vi "VI_unlock.vi"(6 "Verify salt (T)":bool=TRUE, 7 "Remove lib password (T)":bool=TRUE, 8 "error in (no error)":errorcluster, 9 "New Password (\"\")":string, 10 "Output file":path, 11 "Input file":path) -> (0 "error out":errorcluster, 1 "Hash1 salt":string, 2 "Icon":picture, 3 "Version string":string, 4 "Bruteforced salt":bool)   [LabVIEW 2023]
uses:
  <vilib>/Utility/error.llb/Trim Whitespace One-Sided.vi
panel:
  # "(Disable to repair broken BDPW hashes)"
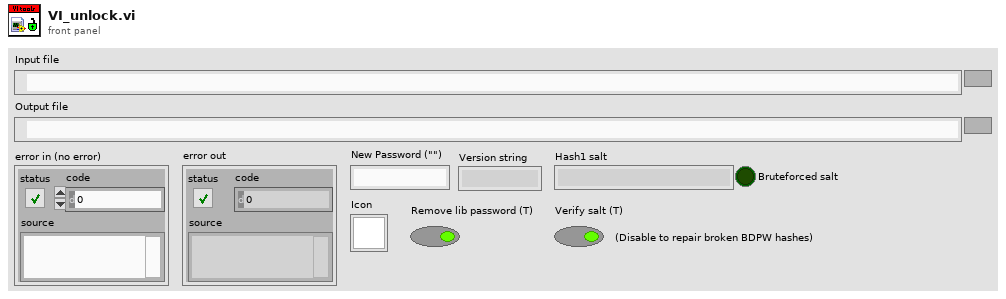
[diagram p1: front panel]
types:
  T1 = cluster{"Major":u8, "Minor":u8, "Fix":u8, "Build":u8}
  T2 = enum16{"open", "replace", "create", "open or create", "replace or create", "replace or create with confirmation"}
  T3 = map{string, cluster{"Offset":i32, "Data":string}}
  T4 = cluster{"Hash1 raw (no salt)":string, "Hash1 (MD5)":string, "VIType":u16}
  T5 = cluster{"version":u32, "Flags":u32, "viFlags2":u32, "viFlags0C":u32, "viFlags10":u32, "buttonsHidden":u16, "frontpFlags":u16, "instrState":u32, "execState":u32, "execPrio":u16, "viType":u16, "prefExecSyst":i32, "field28":u32, "field2C":u32, "field30":u32, "viSignatureHi":u64, "viSignatureLo":u64, "alignGridFP":u32, "alignGridBD":u32, "field4C":u16, "ctrlIndStyle":u16, "field50_md5Hi":u64, "field50_md5Lo":u64, "libHi":u64, "libLo":u64}
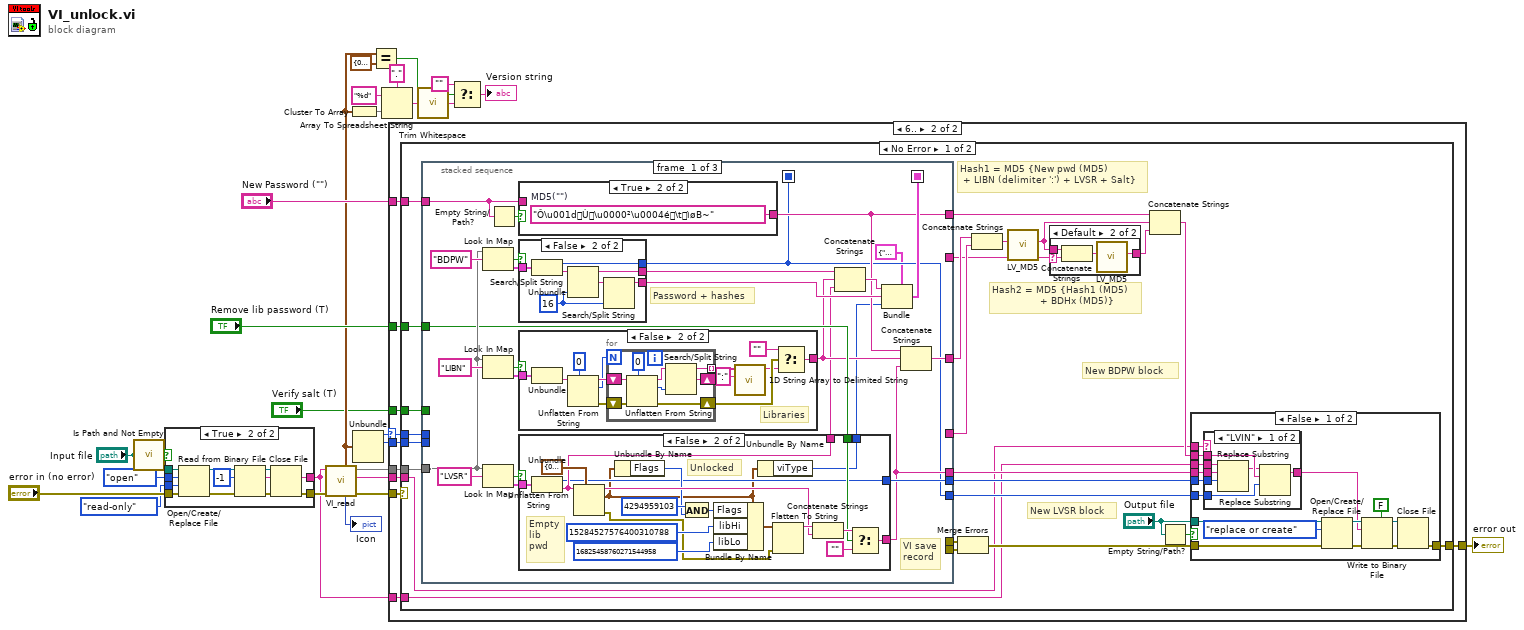
[diagram p0: block diagram]
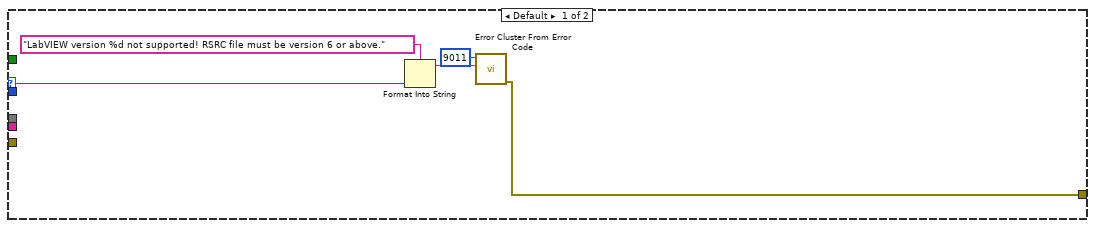
[diagram p2: hidden frame]
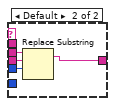
[diagram p4: hidden frame]
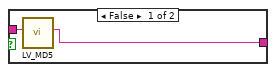
[diagram p6: hidden frame]
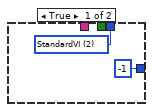
[diagram p7: hidden frame]
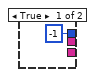
[diagram p9: hidden frame]
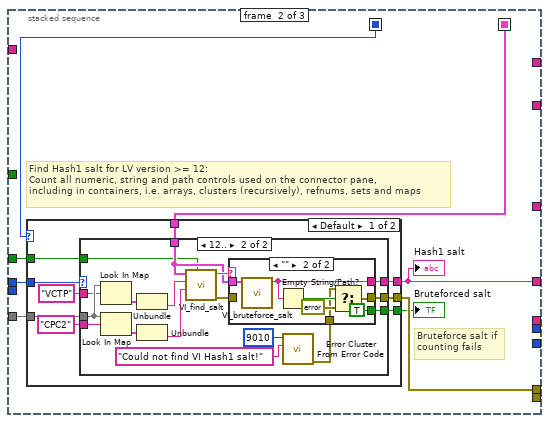
[diagram p10: hidden frame]
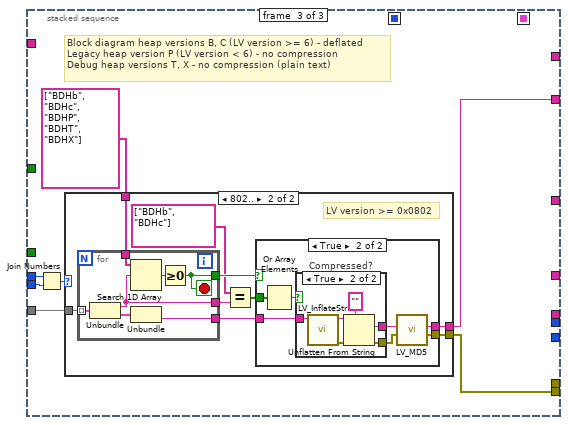
[diagram p14: hidden frame]
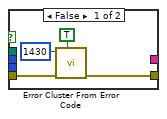
[diagram p19: hidden frame]
diagram:
  n1 = call <vilib>:"Is Path and Not Empty.vi"("path"="Input file") -> ("Is Path and Not Empty?"=w19:bool)  [unwired: 4 in]
  n2 = case "Empty?" shown="True" w19 {
    tunnel: "error in (no error)" -> [w31 w42]
    tunnel: "Input file" -> [_ w41]
    tunnel: [w28 w32] -> w27
    tunnel: enum16{"read/write", "read-only", "write-only"}."read-only" ("access (0:read/write)") -> [_ w40]
    tunnel: T2."open" ("operation (0:open)") -> [_ w39]
    tunnel: [_ w35] -> w5
    frame False {
      n3 = call <vilib>:"Error Cluster From Error Code.vi"("show call chain? (False)"=TRUE, "error in (no error)"=w31, "error code (0)"=1430) -> ("error out"=w28:errorcluster)  [unwired: 6 in]
    }
    frame True {
      n4 = Open/Create/Replace File(file path (use dialog)=w41, error in=w42, operation (0:open)=w39, access (0:read/write)=w40) -> (refnum out=w37:refnum<file>, error out=w38:errorcluster)  [unwired: 2 in, 1 out]
      n5 = Read from Binary File(8:w38, 10:-1 ("count (1)"), 11:w37) -> (0:w33:errorcluster, 2:w35:string, 3:w34:refnum<file>)  [unwired: 3 in, 1 out]
      n6 = Close File(refnum=w34, error in=w33) -> (error out=w32:errorcluster)  [unwired: 1 out]
    }
  }
  n7 = call "VI_read.vi"("error in (no error)"=w27, "File bytestream"=w5) -> ("error out"=w23:errorcluster, "Resource type"=w18:string, "Blocks"=w21:T3, "Icon"=→"Icon":picture, "Version"=w4:T1)  [unwired: 5 in]
  n8 = Cluster To Array(cluster=w4) -> (array=w12:u8[])
  n9 = Unbundle(w4) -> ("Major"=w3:u8, "Minor"=w2:u8)  [unwired: 2 out]
  n10 = Equal?(x=w4, y=T1 {"Major"=0, "Minor"=0, "Fix"=0, "Build"=0}) -> (x = y?=w10:bool)
  n11 = Array To Spreadsheet String(delimiter (Tab)=".", array=w12, 3:"%d" ("format string")) -> (spreadsheet string=w13:string)
  n12 = case shown="6.." w3 {
    selector: w3 -> [w45 w50]
    tunnel: w23 -> [_ w57]
    tunnel: [w43 w56] -> w22
    tunnel: w21 -> [_ w55]
    tunnel: w18 -> [_ w54]
    tunnel: "New Password (\"\")" -> [_ w53]
    tunnel: "Remove lib password (T)" -> [_ w52]
    tunnel: w5 -> [_ w51]
    tunnel: w2 -> [_ w49]
    tunnel: "Verify salt (T)" -> [_ w48]
    frame Default {
      n13 = Format Into String(format string="LabVIEW version %d not supported! RSRC file must be version 6 or above.", w45) -> (resulting string=w44:string)  [unwired: 2 in, 1 out]
      n14 = call <vilib>:"Error Cluster From Error Code.vi"("error message (\"\")"=w44, "error code (0)"=9011) -> ("error out"=w43:errorcluster)  [unwired: 7 in]
    }
    frame 6.. {
      n15 = case shown="No Error" w57 {
        selector: w57 -> [_ w272]
        tunnel: w55 -> [w71 _]
        tunnel: w54 -> [w61 _]
        tunnel: [w62 w272] -> w56
        tunnel: w50 -> [w66 _]
        tunnel: w53 -> [w70 _]
        tunnel: w52 -> [w69 _]
        tunnel: w51 -> [w60 _]
        tunnel: w49 -> [w59 _]
        tunnel: w48 -> [w58 _]
        frame No Error {
          # "New BDPW block"
          # "New LVSR block"
          # "Hash2 = MD5 {Hash1 (MD5)\n                + BDHx (MD5)}"
          # "Hash1 = MD5 {New pwd (MD5)\n + LIBN (delimiter ':') + LVSR + Salt}"
          n16 = stacked-sequence {
            seq-local: [w122 _ _] -> [_ w197 _]
            seq-local: [w117 _ _] -> [_ w193 _]
            tunnel: [_ w195 _] -> w76
            tunnel: w70 -> [w125 _ _]
            tunnel: [_ _ w241] -> w65
            tunnel: [w127 _ _] -> w78
            tunnel: [w120 _ _] -> w77
            tunnel: [w117 _ _] -> w64
            tunnel: [_ _ w240] -> w81
            tunnel: w71 -> [w132 w196 w239]
            tunnel: w69 -> [w128 _ _]
            tunnel: [w119 _ _] -> w68
            tunnel: [w118 _ _] -> w67
            tunnel: w66 -> [_ w199 w237]
            tunnel: [_ w198 _] -> w82
            tunnel: w59 -> [_ _ w236]
            tunnel: w58 -> [_ w192 _]
            frame #0 {
              # "VI save\nrecord"
              # "Password + hashes"
              n17 = Look In Map(map=w132, key="BDPW") -> (key not found?=w138:bool, value=w137:cluster{"Offset":i32, "Data":string})  [unwired: 1 in]
              n18 = Look In Map(map=w132, key="LIBN") -> (key not found?=w135:bool, value=w134:cluster{"Offset":i32, "Data":string})  [unwired: 1 in]
              n19 = Look In Map(map=w132, key="LVSR") -> (key not found?=w130:bool, value=w129:cluster{"Offset":i32, "Data":string})  [unwired: 1 in]
              n20 = Empty String/Path?(string/path=w125) -> (empty?=w126:bool)
              n21 = case shown="True" w126 {
                tunnel: w125 -> [w141 _]
                tunnel: [w140 w142] -> w119
                frame False {
                  n22 = call "LV_MD5.vi"("Input string"=w141) -> ("MD5 digest (16-bytes)"=w140:string)  [unwired: 9 in, 1 out]
                }
                frame True {
                  w142 = "Ô\u001dÙ\u0000²\u0004é\tìøB~"  # MD5("")
                }
              }
              n23 = case "Has BDPW?" shown="False" w138 {
                tunnel: w137 -> [_ w191]
                tunnel: [-1 ("Offset") w190] -> w117
                tunnel: [_ w186] -> w131
                tunnel: [_ w185] -> w123
                frame True {
                }
                frame False {
                  w187 = 16 ("offset (0)")
                  n24 = Unbundle(w191) -> ("Offset"=w190:i32, "Data"=w189:string)
                  n25 = Search/Split String(string=w189, offset (0)=w187) -> (substring before match=w186:string, match + rest of string=w188:string)  [unwired: 1 in, 1 out]
                  n26 = Search/Split String(string=w188, offset (0)=w187) -> (substring before match=w185:string)  [unwired: 1 in, 2 out]
                }
              }
              n27 = case "Has LIBN?" shown="False" w135 {
                tunnel: w134 -> [_ w171]
                tunnel: [_ w164] -> w121
                frame True {
                }
                frame False {
                  # "Libraries"
                  n28 = Unbundle(w171) -> ("Data"=w170:string)  [unwired: 1 out]
                  n29 = Unflatten From String(type=0 ("I32"), binary string=w170) -> (rest of the binary string=w173:string, value=w172:i32, error out=w174:errorcluster)  [unwired: 3 in]
                  n30 = for {
                    N: w172 -> [_]
                    shift-right: [w177] -> _
                    shift-left: w173 -> [w181]
                    shift-right: [w178] -> w167
                    shift-left: w174 -> [w182]
                    tunnel: [w176] -> w169 mode=indexing
                    n31 = Unflatten From String(type=u8 0 ("U8"), binary string=w181, error in (no error)=w182) -> (rest of the binary string=w180:string, value=w179:u8, error out=w178:errorcluster)  [unwired: 2 in]
                    n32 = Search/Split String(string=w180, offset (0)=w179) -> (substring before match=w176:string, match + rest of string=w177:string)  [unwired: 1 in, 1 out]
                  }
                  n33 = call <vilib>:"1D String Array to Delimited String.vi"("delimiter"=":", "string array"=w169) -> ("delimited string"=w166:string)  [unwired: 9 in]
                  n34 = Select(t="", s=w167, f=w166) -> (s? t:f=w164:string)
                }
              }
              n35 = case "Has LIBN?" shown="False" w130 {
                tunnel: w129 -> [_ w153]
                tunnel: [_ w149] -> w118
                tunnel: w128 -> [_ w151]
                tunnel: [-1 ("Offset") w147] -> w127
                tunnel: [_ w152] -> w116
                tunnel: [w143 w145] -> w115
                frame True {
                  w143 = u16 2 items=["DialogVI", "ProbeVI", "StandardVI", "ClipboardVI", "GlobalVI", "HierarchyVI", "ControlVI", "ConfigVI", "PxCallerVI", "PxCalleeVI", "SubSystemVI", "PolyVI", "FacadeVI", "MethodVI", "StatechartVI"] ("VIType")
                }
                frame False {
                  # "Unlocked"
                  # "Empty\nlib\npwd"
                  n36 = Unbundle(w153) -> ("Offset"=w147:i32, "Data"=w152:string)
                  n37 = Unflatten From String(type=T5 {"version"=0, "Flags"=0, "viFlags2"=0, "viFlags0C"=0, "viFlags10"=0, "buttonsHidden"=0, "frontpFlags"=0, "instrState"=0, "execState"=0, "execPrio"=0, "viType"=0, "prefExecSyst"=0, "field28"=0, "field2C"=0, "field30"=0, "viSignatureHi"=0, "viSignatureLo"=0, "alignGridFP"=0, "alignGridBD"=0, "field4C"=0, "ctrlIndStyle"=0, "field50_md5Hi"=0, "field50_md5Lo"=0, "libHi"=0, "libLo"=0} ("LVSR"), binary string=w152) -> (rest of the binary string=w160:string, value=w146:T5, error out=w148:errorcluster)  [unwired: 3 in]
                  n38 = Unbundle By Name(w146) -> ("Flags"=w150:u32)
                  n39 = And(x=u32 4294959103 ("Unlocked"), y=w150) -> (x .and. y?=w154:u32)
                  n40 = Bundle By Name(cluster=w146, "Flags"=w154, "libHi"=u64 15284527576400310788 ("libpass_md5Hi"), "libLo"=u64 16825458760271544958 ("libpass_md5Lo")) -> (w159:T5)
                  n41 = Unbundle By Name(w146) -> ("viType"=w145:u16)
                  n42 = Flatten To String(anything=w159, error in (no error)=w148) -> (data string=w161:string)  [unwired: 2 in, 2 out]
                  n43 = Concatenate Strings(w161, w160) -> (w163:string)
                  n44 = Select(t=w163, s=w151, f="") -> (s? t:f=w149:string)
                }
              }
              n45 = Concatenate Strings(w131, w121, w116) -> (w124:string)
              n46 = Bundle(cluster=T4 {"Hash1 raw (no salt)"="", "Hash1 (MD5)"="", "VIType"=2} ("output cluster"), "Hash1 raw (no salt)"=w124, "Hash1 (MD5)"=w123, "VIType"=w115) -> (w122:T4)
              n47 = Concatenate Strings(w119, w121, w118) -> (w120:string)
            }
            frame #1 {
              # "Bruteforce salt if\ncounting fails"
              # "Find Hash1 salt for LV version >= 12:\nCount all numeric, string and path controls used on the connector pane,\nincluding in containers, i.e. arrays, clusters (recursively), refnums, sets and maps"
              n48 = case shown="Default" w193 {
                tunnel: [w208 _] -> w195
                tunnel: w199 -> [w205 _]
                tunnel: [w207 _] -> w198
                tunnel: w197 -> [w206 _]
                tunnel: w196 -> [w204 _]
                tunnel: [w202 _] -> w194
                tunnel: w192 -> [w200 _]
                frame Default {
                  n49 = case shown="12.." w205 {
                    tunnel: [_ w220] -> w208
                    tunnel: w206 -> [_ w210]
                    tunnel: [_ w221] -> w207
                    tunnel: w204 -> [_ w215]
                    tunnel: "CPC2" ("key") -> [_ w224]
                    tunnel: [_ w216] -> w202
                    tunnel: "VCTP" ("key") -> [_ w214]
                    tunnel: w200 -> [_ w209]
                    frame Default {
                    }
                    frame 12.. {
                      n50 = Look In Map(map=w215, key=w214) -> (value=w213:cluster{"Offset":i32, "Data":string})  [unwired: 1 in, 1 out]
                      n51 = Look In Map(map=w215, key=w224) -> (value=w225:cluster{"Offset":i32, "Data":string})  [unwired: 1 in, 1 out]
                      n52 = Unbundle(w213) -> ("Data"=w212:string)  [unwired: 1 out]
                      n53 = Unbundle(w225) -> ("Data"=w211:string)  [unwired: 1 out]
                      n54 = call "VI_find_salt.vi"("Verify salt (T)"=w209, "CPC2 block"=w211, "VCTP block"=w212, "Hashes"=w210) -> ("error out"=w222:errorcluster, "Salt"=w223:string)  [unwired: 6 in]
                      n55 = call <vilib>:"Error Cluster From Error Code.vi"("error message (\"\")"="Could not find VI Hash1 salt!" ("error message (\"\")"), "error code (0)"=9010) -> ("error out"=w217:errorcluster)  [unwired: 7 in]
                      n56 = case shown="\"\"" w223 {
                        selector: w223 -> [w226 _]
                        tunnel: [w227 w229] -> w221
                        tunnel: w222 -> [w227 _]
                        tunnel: [w226 w233] -> w220
                        tunnel: w210 -> [_ w234]
                        tunnel: w217 -> [_ w230]
                        tunnel: [_ TRUE] -> w216
                        frame Default {
                        }
                        frame "" {
                          n57 = call "VI_bruteforce_salt.vi"("Hashes"=w234) -> ("Salt"=w233:string)  [unwired: 10 in]
                          n58 = Empty String/Path?(string/path=w233) -> (empty?=w232:bool)
                          n59 = Select(t=w230, s=w232, f=errorcluster {"status"=FALSE, "code"=0, "source"=""}) -> (s? t:f=w229:errorcluster)
                        }
                      }
                    }
                  }
                }
                frame ..-1 {
                  # "No BDPW block (global variables, controls etc.)"
                }
              }
              "Hash1 salt" <- w195
              "Bruteforced salt" <- w194
            }
            frame #2 {
              # "Block diagram heap versions B, C (LV version >= 6) - deflated\nLegacy heap version P (LV version < 6) - no compression\nDebug heap versions T, X - no compression (plain text)"
              n60 = Join Numbers(hi=w237, lo=w236) -> ((hi.lo)=w238:u16)
              n61 = case shown="802.." w238 {
                tunnel: [_ w249] -> w241
                tunnel: [_ w248] -> w240
                tunnel: w239 -> [_ w247]
                tunnel: string[] ["BDHb", "BDHc", "BDHP", "BDHT", "BDHX"] -> [_ w242]
                frame Default {
                  # "LV version < 8.2: No Hash2"
                }
                frame 2050.. {
                  # "LV version >= 0x0802"
                  n62 = for {
                    tunnel: w247 -> [w255] mode=indexing
                    tunnel: [w254] -> w246
                    tunnel: [w252] -> w245
                    tunnel: [w256] -> w244
                    tunnel: w242 -> [w251]
                    stop <- w252 stop-if-true
                    n63 = Unbundle(w255) -> (w254:string, "value"=w257:cluster{"Offset":i32, "Data":string})
                    n64 = Search 1D Array(1D array=w251, element=w254) -> (index of element=w253:i32)  [unwired: 1 in]
                    n65 = Unbundle(w257) -> ("Data"=w256:string)  [unwired: 1 out]
                    n66 = Greater Or Equal To 0?(x=w253) -> (x >= 0?=w252:bool)
                  }
                  n67 = Equal?(x=string[] ["BDHb", "BDHc"], y=w246) -> (x = y?=w250:bool[])
                  n68 = case shown="True" w245 {
                    tunnel: w250 -> [_ w264]
                    tunnel: w244 -> [_ w262]
                    tunnel: [_ w259] -> w248
                    tunnel: [_ w258] -> w249
                    frame False {
                    }
                    frame True {
                      n69 = Or Array Elements(Boolean array=w264) -> (logical OR=w263:bool)
                      n70 = case "Compressed?" shown="True" w263 {
                        tunnel: w262 -> [w265 w269]
                        tunnel: [_ w271] -> w260
                        tunnel: [w265 w270] -> w261
                        frame False {
                        }
                        frame True {
                          n71 = call "LV_InflateStr.vi"("Deflated string with size header"=w269) -> ("error out"=w267:errorcluster, "Inflated string"=w268:string)  [unwired: 9 in]
                          n72 = Unflatten From String(type="", binary string=w268, error in (no error)=w267) -> (value=w270:string, error out=w271:errorcluster)  [unwired: 2 in, 1 out]
                        }
                      }
                      n73 = call "LV_MD5.vi"("error in (no error)"=w260, "Input string"=w261) -> ("error out"=w259:errorcluster, "MD5 digest (16-bytes)"=w258:string)  [unwired: 8 in]
                    }
                  }
                }
              }
            }
          }
          n74 = Merge Errors(w82, w81) -> (w63:errorcluster)
          n75 = Concatenate Strings(w77, w76) -> (w74:string)
          n76 = call "LV_MD5.vi"("Input string"=w74) -> ("MD5 digest (16-bytes)"=w73:string)  [unwired: 9 in, 1 out]
          n77 = case shown="Default" w65 {
            selector: w65 -> [_ w83]
            tunnel: w73 -> [_ w86]
            tunnel: [_ w84] -> w72
            frame "" {
            }
            frame Default {
              n78 = Concatenate Strings(w86, w83) -> (w85:string)
              n79 = call "LV_MD5.vi"("Input string"=w85) -> ("MD5 digest (16-bytes)"=w84:string)  [unwired: 9 in, 1 out]
            }
          }
          n80 = Concatenate Strings(w68, w73, w72) -> (w75:string)
          n81 = Empty String/Path?(string/path="Output file") -> (empty?=w80:bool)
          n82 = case shown="False" w80 {
            tunnel: [w95 _] -> w62
            tunnel: "Output file" -> [w94 _]
            tunnel: w60 -> [w93 _]
            tunnel: w61 -> [w92 _]
            tunnel: w64 -> [w87 _]
            tunnel: w75 -> [w91 _]
            tunnel: w78 -> [w90 _]
            tunnel: w67 -> [w89 _]
            tunnel: w63 -> [w88 _]
            frame False {
              n83 = case shown="\"LVIN\"" w92 {
                tunnel: w93 -> [w105 w113]
                tunnel: [w103 w110] -> w96
                tunnel: w91 -> [w109 _]
                tunnel: w90 -> [w107 w111]
                tunnel: w89 -> [w108 w112]
                tunnel: w87 -> [w106 _]
                frame "LVIN" {
                  n84 = Replace Substring(3:w107, 4:w108, 5:w105) -> (1:w104:string)  [unwired: 1 in, 1 out]
                  n85 = Replace Substring(3:w106, 4:w109, 5:w104) -> (1:w103:string)  [unwired: 1 in, 1 out]
                }
                frame Default {
                  n86 = Replace Substring(3:w111, 4:w112, 5:w113) -> (1:w110:string)  [unwired: 1 in, 1 out]
                }
              }
              n87 = Open/Create/Replace File(file path (use dialog)=w94, error in=w88, operation (0:open)=T2."replace or create") -> (refnum out=w98:refnum<file>, error out=w101:errorcluster)  [unwired: 1 in, 3 out]
              n88 = Write to Binary File(file (use dialog)=w98, data=w96, error in=w101, 5:FALSE ("prepend array or string size? (T)")) -> (refnum out=w100:refnum<file>, error out=w99:errorcluster)  [unwired: 2 in, 1 out]
              n89 = Close File(refnum=w100, error in=w99) -> (error out=w95:errorcluster)  [unwired: 1 out]
            }
            frame True {
            }
          }
        }
        frame Default {
        }
      }
    }
  }
  "error out" <- w22
  n90 = call <vilib>:"Trim Whitespace.vi"("string"=w13) -> ("trimmed string"=w9:string)  [unwired: 1 in]
  n91 = Select(t="", s=w10, f=w9) -> (s? t:f=→"Version string":string)
